vi "Send Command.vi"(8 "error in":errorcluster, 9 "Value":variant, 10 "Command":string, 11 "AnalogInput in":refnum<class "AnalogInput.lvclass">) -> (0 "error out":errorcluster, 3 "AnalogInput out":refnum<class "AnalogInput.lvclass">)   [LabVIEW 2019, in "AnalogInput.lvlib" / "AnalogInput.lvclass"]
uses:
  Library/AnalogInput.lvclass
  C:/Users/Public/Documents/Development/builds/Engine/Engine.lvlibp/Project/Engine.lvclass
  Custom Controls/User Trigger Settings.ctl
  Custom Controls/Trigger_Slope.ctl
  AnalogInput Messages/Write User Trigger Settings Msg/Write User Trigger Settings Msg.lvclass/Write User Trigger Settings Msg.ctl
  AnalogInput Messages/Write Trigger Source Msg/Write Trigger Source Msg.lvclass/Write Trigger Source Msg.ctl
  builds/Engine/Engine.lvlibp/Accessors/Read Self Q.vi
  builds/Engine/Actor Framework.lvlibp/1abvi3w/vi.lib/ActorFramework/Message Enqueuer/Enqueue.vi
  builds/Engine/Actor Framework.lvlibp/1abvi3w/vi.lib/ActorFramework/Message Enqueuer/Message Enqueuer.lvclass
  AnalogInput Messages/Write User Trigger Settings Msg/Write User Trigger Settings Msg.lvclass
  AnalogInput Messages/Write Trigger Source Msg/Write Trigger Source Msg.lvclass
  builds/Instruments/Instruments.lvlibp/Instruments Messages/Take Snapshot Msg/Take Snapshot Msg.lvclass
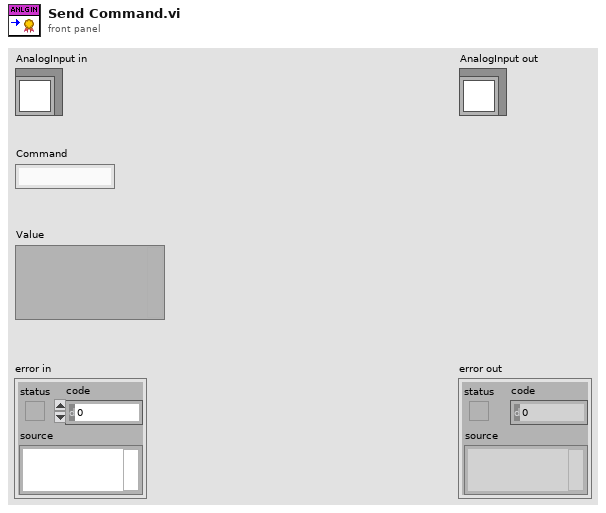
[diagram p1: front panel]
types:
  T1 = typedef "AnalogInput.lvlib/AnalogInput.lvclass/User Trigger Settings.ctl" = cluster{"Timeout":dbl, "Level":dbl, "Slope":T2, "samples per channel":i32, "Sample Rate (10k)":dbl, "pretrigger samples":u32}
  T2 = typedef "AnalogInput.lvlib/AnalogInput.lvclass/Trigger_Slope.ctl" = enum16{"Rising", "Falling"}
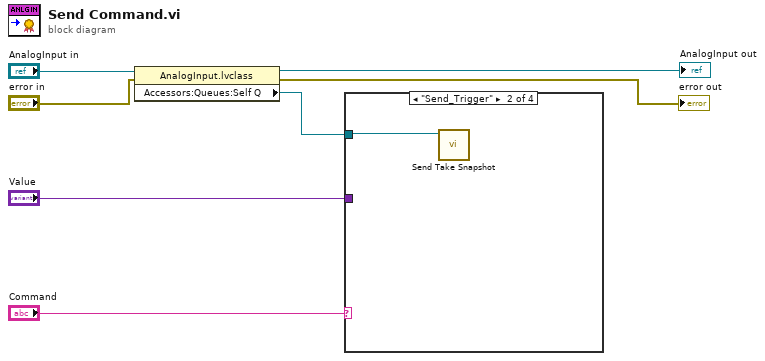
[diagram p0: block diagram]
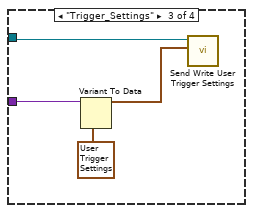
[diagram p3: hidden frame]
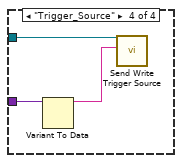
[diagram p4: hidden frame]
diagram:
  n1 = property class="AnalogInput.lvclass"(reference="AnalogInput in", error in="error in") -> (reference out=→"AnalogInput out":refnum<class "AnalogInput.lvclass">, error out=→"error out":errorcluster, "Accessors:Queues:Self Q"=w2:refnum<class "Message Enqueuer.lvclass">)
  n2 = case shown="\"Send_Trigger\"" "Command" {
    tunnel: w2 -> [_ w8 w10 w15]
    tunnel: "Value" -> [_ _ w12 w13]
    frame "False", Default {
    }
    frame "Send_Trigger" {
      n3 = call "Send Take Snapshot.vi"("Message Enqueuer"=w8) -> ()  [unwired: 9 in, 2 out]
    }
    frame "Trigger_Settings" {
      n4 = Variant To Data(type=T1 {"Timeout"=0.0, "Level"=0.0, "Slope"=enum."Falling", "samples per channel"=100, "Sample Rate (10k)"=10000.0, "pretrigger samples"=500} ("User Trigger Settings"), Variant=w12) -> (data=w9:T1)  [unwired: 1 in, 1 out]
      n5 = call "Send Write User Trigger Settings.vi"("User Trigger Settings"=w9, "Message Enqueuer"=w10) -> ()  [unwired: 8 in, 2 out]
    }
    frame "Trigger_Source" {
      n6 = Variant To Data(Variant=w13) -> (data=w14:string)  [unwired: 2 in, 1 out]
      n7 = call "Send Write Trigger Source.vi"("Trigger Source"=w14, "Message Enqueuer"=w15) -> ()  [unwired: 8 in, 2 out]
    }
  }
